vi "DotNETCam_SendUiEvent.vi"(6 "UiEventNames":T1, 8 "ErrorIn":errorcluster, 11 "DotNETCamIn":refnum<class "DotNETCam.lvclass">) -> (0 "ErrorOut":errorcluster, 3 "DotNETCamOut":refnum<class "DotNETCam.lvclass">)   [LabVIEW 2021, in "DotNETCam.lvclass"]
uses:
  DotNETCam.lvclass
  DotNETCam_UiCallBackEvents.ctl
  DotNETCam.lvclass/DotNETCam.ctl
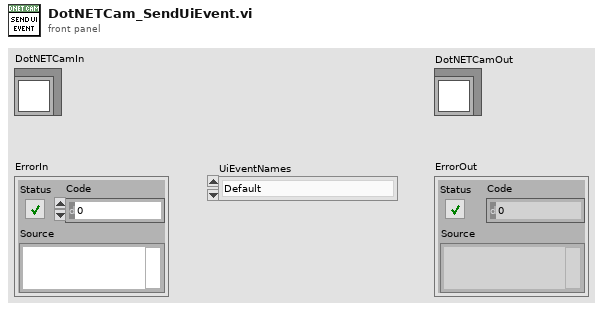
[diagram p1: front panel]
types:
  T1 = typedef "DotNETCam.lvclass/DotNETCam_UiCallBackEvents.ctl" = enum16{"Default", "PersistentDataUpdated", "Worker 1: Do Something"}
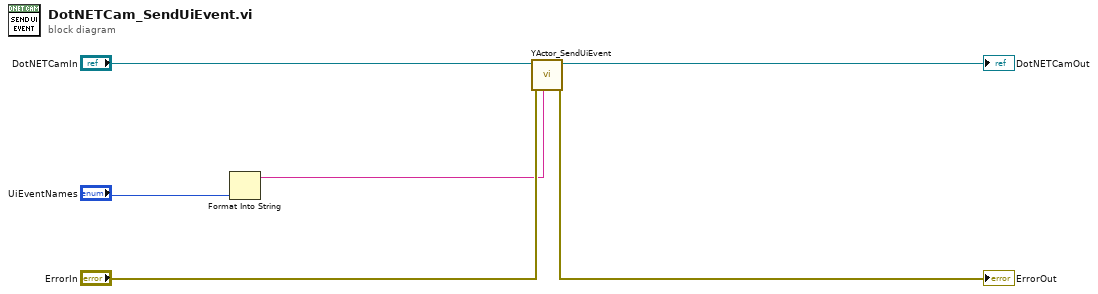
[diagram p0: block diagram]
diagram:
  n1 = Format Into String("UiEventNames") -> (resulting string=w1:string)  [unwired: 3 in, 1 out]
  n2 = call-dynamic "YActor_SendUiEvent.vi"("Event"=w1, "ErrorIn"="ErrorIn", "YActorIn"="DotNETCamIn") -> ("ErrorOut"=→"ErrorOut":errorcluster, "YActorOut"=→"DotNETCamOut":refnum<class "DotNETCam.lvclass">)  [unwired: 7 in]
